vi "rvc Scale Matrix.vi"(10 "scale (1)":dbl, 11 "end effector transform":T1) -> (3 "transform":T1)   [LabVIEW 2014]
uses:
  <vilib>/Analysis/Matrix/Datatypes/RealMatrix.ctl
  <vilib>/robotics/Kinematics/NI_Kinematics.lvlib
  <vilib>/Analysis/Matrix/NI_Matrix.lvlib
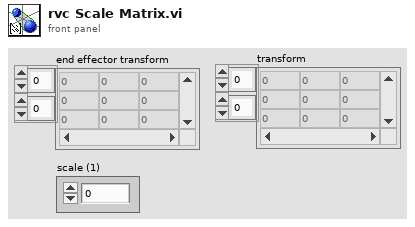
[diagram p1: front panel]
types:
  T1 = typedef "NI_Matrix.lvlib/RealMatrix.ctl" = dbl[][]
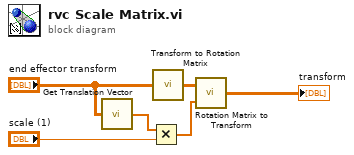
[diagram p0: block diagram]
diagram:
  n1 = call <vilib>:"Get Translation Vector.vi"("transform"="end effector transform") -> ("translation vector"=w4:dbl[])
  n2 = Multiply(x=w4, y="scale (1)") -> (x*y=w3:dbl[])
  n3 = call <vilib>:"Transform to Rotation Matrix.vi"("transform"="end effector transform") -> ("rotation matrix"=w2:T1)
  n4 = call <vilib>:"Rotation Matrix to Transform.vi"("translation vector"=w3, "rotation matrix"=w2) -> ("transform"=→"transform":T1)
